vi "WaitForNextCleanMinute.vi"() -> (0 "Seconds to wait":dbl)   [LabVIEW 2017]
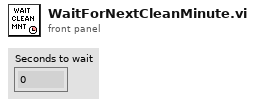
[diagram p1: front panel]
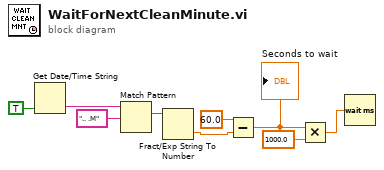
[diagram p0: block diagram]
diagram:
  n1 = Get Date/Time String(want seconds? (F)=TRUE) -> (time string=w2:string)  [unwired: 2 in, 1 out]
  n2 = Match Pattern(string=w2, regular expression=".. .M") -> (match substring=w1:string)  [unwired: 1 in, 3 out]
  n3 = Fract/Exp String To Number(string=w1) -> (number=w7:dbl)  [unwired: 3 in, 1 out]
  n4 = Subtract(x=60.0, y=w7) -> (x-y=w6:dbl)
  "Seconds to wait" <- w6
  n5 = Multiply(x=w6, y=1000.0) -> (x*y=w9:dbl)
  n6 = Wait (ms)(milliseconds to wait=w9) -> ()  [unwired: 1 out]
